vi "Delete Topics.vi"(8 "error in (no error)":errorcluster, 11 "Array of Topics to be Deleted":string[](array[string])) -> (0 "error out":errorcluster)   [LabVIEW 2014]
uses:
  <vilib>/National Instruments/NI Amazon Web Services (AWS) Toolkit for LabVIEW/SNS/VI Source/Response Typedefs/ListTopicsResult.ctl
  <vilib>/National Instruments/NI Amazon Web Services (AWS) Toolkit for LabVIEW/S3/vi source/Typedefs/AMZ_S3_AWS Credentials.ctl
  <vilib>/National Instruments/NI Amazon Web Services (AWS) Toolkit for LabVIEW/AWS Core Lib/VI Source/Typedefs/AWS_Region.ctl
  <vilib>/National Instruments/NI Amazon Web Services (AWS) Toolkit for LabVIEW/SNS/VI Source/AWS SNS Class/AWS_SNS.lvclass
  <vilib>/National Instruments/NI Amazon Web Services (AWS) Toolkit for LabVIEW/S3/vi source/LV Interface for Amazon S3.lvlib
  <vilib>/National Instruments/NI Amazon Web Services (AWS) Toolkit for LabVIEW/AWS Core Lib/VI Source/AWS_Core.lvlib
  <vilib>/National Instruments/NI Amazon Web Services (AWS) Toolkit for LabVIEW/SNS/VI Source/AWS_SNS.lvlib
panel:
  in  "Topics":string[](array[string])
  out "ListTopic Result":T1
  # "Use this to delete an array of topics"
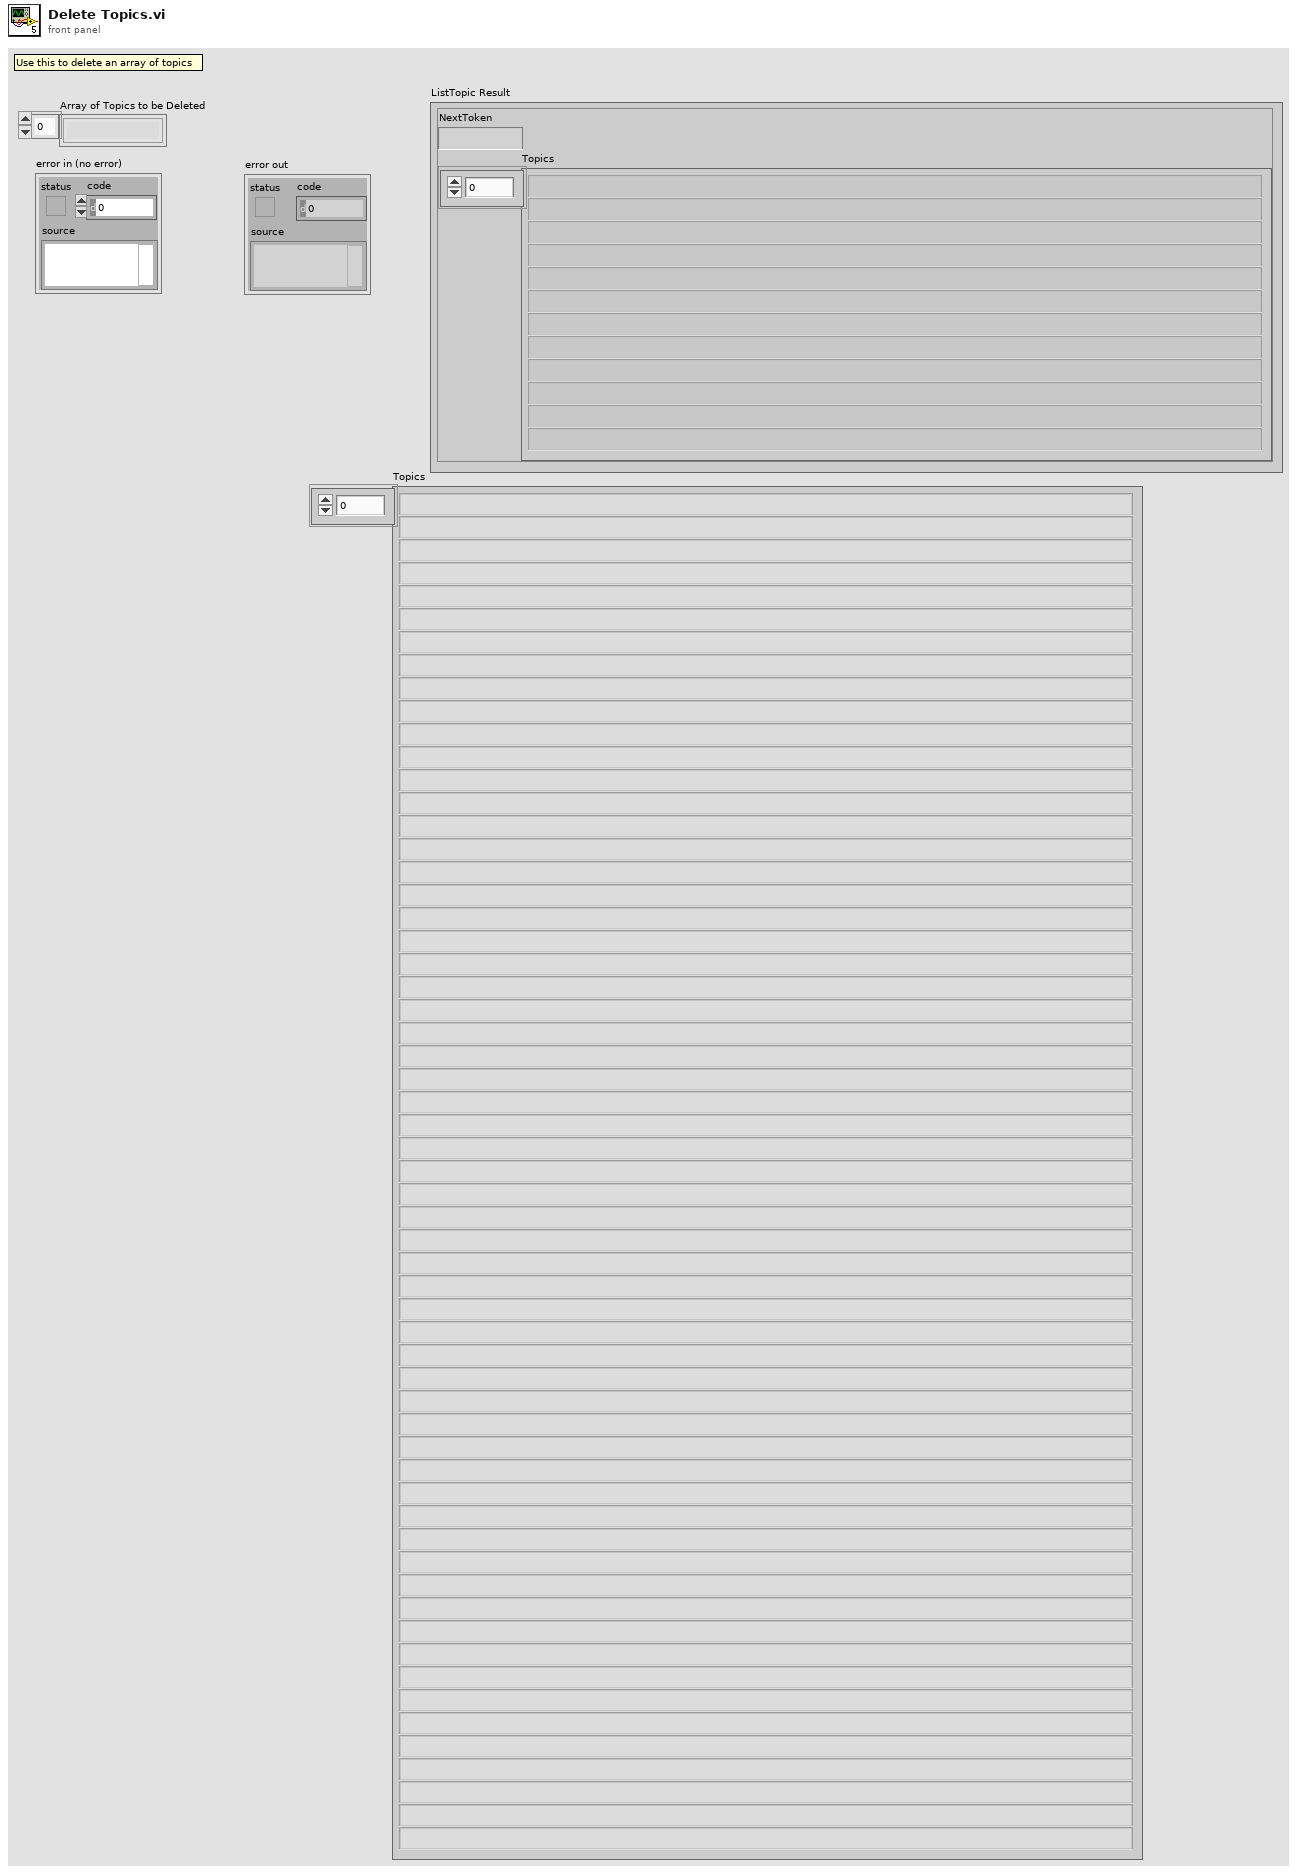
[diagram p1: front panel]
types:
  T1 = typedef "AWS_SNS.lvlib/ListTopicsResult.ctl" = cluster{"NextToken":string, "Topics":string[]}
  T2 = typedef "AWS_Core.lvlib/AWS_Region.ctl" = enum16{"us-east-1"}
  T3 = typedef "LV Interface for Amazon S3.lvlib/AMZ_S3_AWS Credentials.ctl" = cluster{"Access Key":string, "Secret Key":string}
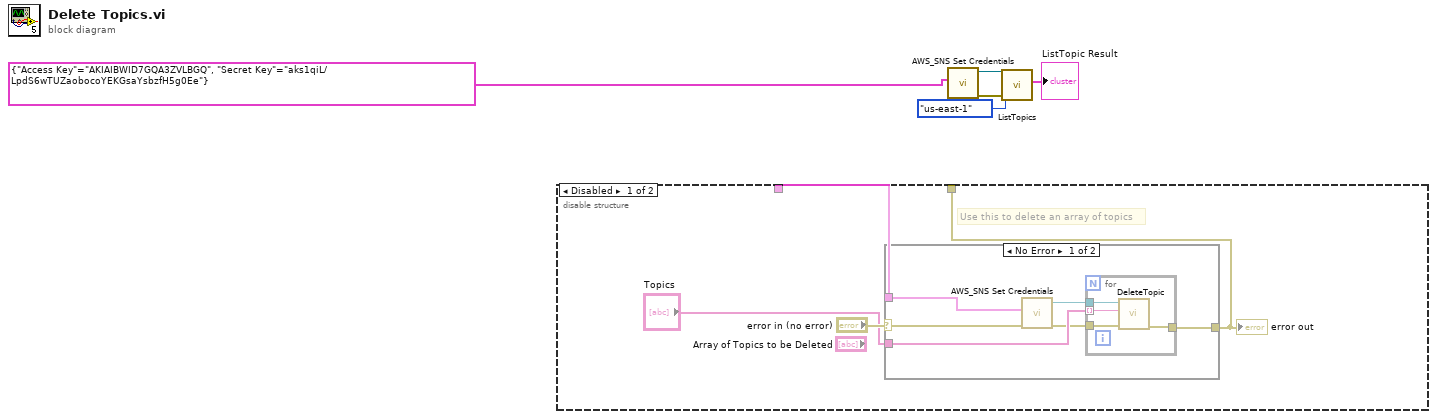
[diagram p0: block diagram]
diagram:
  n1 = disable-structure shown="Disabled" {
    disable-tunnel: _ -> [w7 _]
    disable-tunnel: [w6 _] -> _
    frame Disabled {
      # "Use this to delete an array of topics"
      n2 = case shown="No Error" "error in (no error)" {
        selector: "error in (no error)" -> [w13 w20]
        tunnel: "Topics" -> [w14 _]
        tunnel: [w11 w20] -> w6
        tunnel: w7 -> [w10 _]
        frame No Error {
          n3 = call <vilib>:"AWS_SNS Set Credentials.vi"("error in (no error)"=w13, "AWS Credentials"=w10) -> ("error out"=w12:errorcluster, "AWS_SNS.lvlib:AWS_SNS.lvclass"=w15:refnum<class "AWS_SNS.lvclass">)  [unwired: 8 in]
          n4 = for {
            tunnel: w15 -> [w19]
            tunnel: w14 -> [w18] mode=indexing
            tunnel: w12 -> [w17]
            tunnel: [w16] -> w11
            n5 = call-dynamic "DeleteTopic.vi"("AWS_SNS in"=w19, "TopicArn"=w18, "error in (no error)"=w17) -> ("error out"=w16:errorcluster)  [unwired: 6 in, 1 out]
          }
        }
        frame Error {
        }
      }
      "error out" <- w6
    }
    frame Enabled {
    }
  }
  n6 = call <vilib>:"AWS_SNS Set Credentials.vi"("AWS Credentials"=T3 {"Access Key"="AKIAIBWID7GQA3ZVLBGQ", "Secret Key"="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"} ("AWS Credentials in")) -> ("error out"=w5:errorcluster, "AWS_SNS.lvlib:AWS_SNS.lvclass"=w4:refnum<class "AWS_SNS.lvclass">)  [unwired: 9 in]
  n7 = call <vilib>:"ListTopics.vi"("error in (no error)"=w5, "Region"=AWS_Region."us-east-1", "AWS_SNS in"=w4) -> ("ListTopic Result"=→"ListTopic Result":T1)  [unwired: 6 in, 2 out]
